vi "MCB2400 AI PrjAttrValidator.vi"(5 "Ctl Refnum":refnum<vi>, 9 "Channel Num":u8(ring) items=["143", "144", "145", "146", "147", "148", "149", "150"], 11 "Attributes":T1 {"Programmable Pin Connections" items=["AI0 uses pin P0.23. You cannot use AI0 and pin P0.23 in the same project.", "AI1 uses pin P0.24. You cannot use AI1 and pin P0.24 in the same project. ", "AI2 uses pin P0.25. You cannot use AI2 and pin P0.25 in the same project.", "AI3 uses pin P0.26 (also used by AOUT). You cannot use AI3 and pin P0.26 (or AOUT) in the same project.", "AI4 uses pin P1.30. You cannot use AI4 and pin P1.30 in the same project.", "AI5 uses pin P1.31. You cannot use AI5 and pin P1.31 in the same project.", "AI6 uses pin P0.12. You cannot use AI6 and pin P0.12 in the same project.", "AI7 uses pin P0.13. You cannot use AI7 and pin P0.13 in the same project."]}) -> (3 "Valid?":bool)   [LabVIEW 2011]
uses:
  <vilib>/Embedded/ARM/MCB2400/MCB2400_AI_PrjAttr.ctl
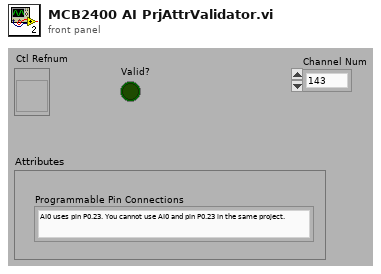
[diagram p1: front panel]
types:
  T1 = typedef "MCB2400_AI_PrjAttr.ctl" = cluster{"Programmable Pin Connections":u16}
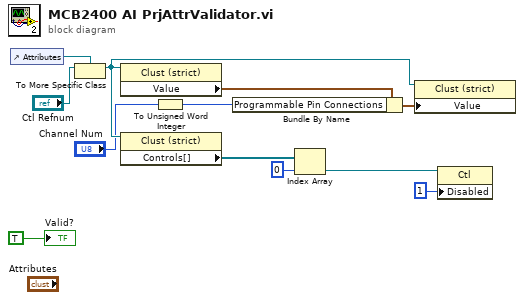
[diagram p0: block diagram]
diagram:
  n1 = control-ref of="Attributes"() -> (w4:refnum<vi>)
  n2 = To More Specific Class(target class=w4, reference="Ctl Refnum") -> (specific class reference=w5:refnum<vi>)  [unwired: 1 in, 1 out]
  n3 = property class="Clust (strict)"(reference=w5) -> ("Value"=w11:cluster{"Programmable Pin Connections":u16})  [unwired: 1 in, 2 out]
  n4 = property class="Clust (strict)"(reference=w5) -> ("Controls[]"=w9:refnum<vi>[])  [unwired: 1 in, 2 out]
  n5 = To Unsigned Word Integer(number="Channel Num") -> (unsigned 16bit integer=w1:u16)
  n6 = Bundle By Name(cluster=w11, "Programmable Pin Connections"=w1) -> (w10:cluster{"Programmable Pin Connections":u16})
  n7 = Index Array(array=w9, index=0) -> (element=w7:refnum<vi>)
  n8 = property class="Clust (strict)"(reference=w5, "Value"=w10) -> ()  [unwired: 1 in, 2 out]
  n9 = property class="Ctl"(reference=w7, "Disabled"=u8 1) -> ()  [unwired: 1 in, 2 out]
  "Valid?" <- TRUE ("Valid?")
